vi "Read currentTimeToObservable_min.vi"(8 "error in (no error)":errorcluster, 11 "Limits in":refnum<class "Limits.lvclass">) -> (0 "error out":errorcluster, 2 "currentTimeToObservable_min":dbl[unit], 3 "Limits out":refnum<class "Limits.lvclass">)   [LabVIEW 2022 SP3, in "TCSDataDefinitions.lvlib" / "TCSPublicStatus.lvlib" / "Limits.lvlib" / "Limits.lvclass"]
uses:
  Limits.lvclass
  Limits.lvclass/Limits.ctl
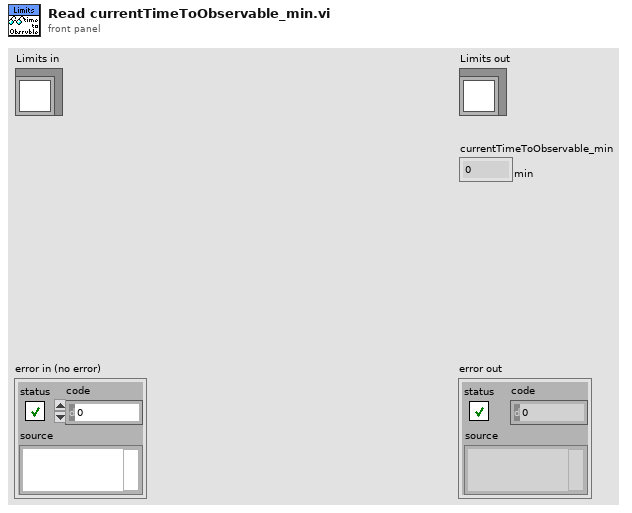
[diagram p1: front panel]
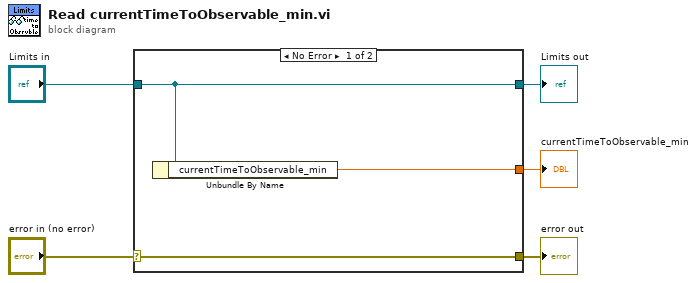
[diagram p0: block diagram]
diagram:
  n1 = case shown="No Error" "error in (no error)" {
    selector: "error in (no error)" -> [w8 w9]
    tunnel: [w8 w9] -> w4
    tunnel: [w7 w10] -> w2
    tunnel: "Limits in" -> [w7 w10]
    tunnel: [w6 _] -> w1
    frame No Error {
      n2 = Unbundle By Name(w7) -> ("currentTimeToObservable_min"=w6:dbl[unit])
    }
    frame Error {
    }
  }
  "error out" <- w4
  "Limits out" <- w2
  "currentTimeToObservable_min" <- w1
